vi "build_version_msg.vi"(4 "error in":errorcluster, 5 "Client version":string, 6 "Client API version":string, 7 "Response JSON":string) -> (0 "error out":errorcluster, 2 "API version":string, 3 "Message":string)   [LabVIEW 2019]
doc: "Builds a message to inform the user the compatibility between simulator and client."
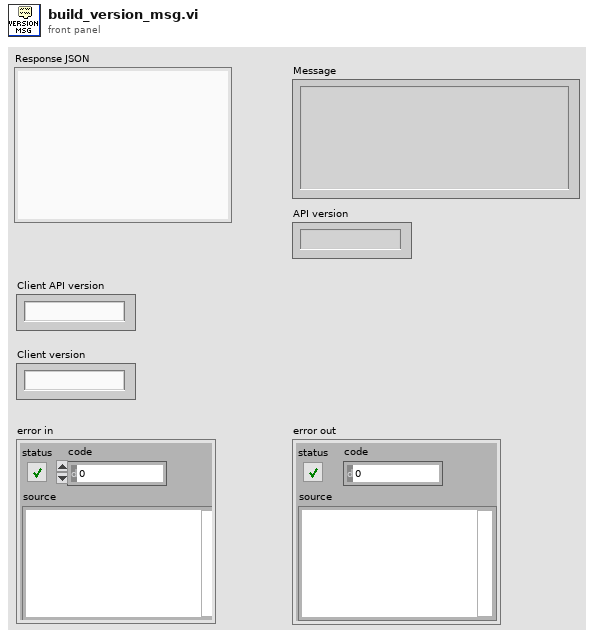
[diagram p1: front panel]
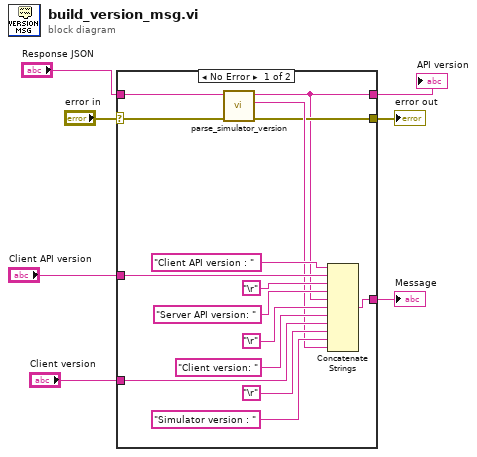
[diagram p0: block diagram]
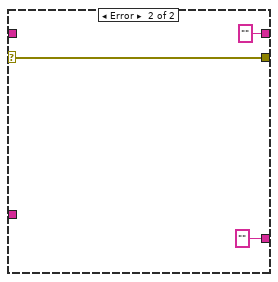
[diagram p2: hidden frame]
diagram:
  n1 = case shown="No Error" "error in" {
    selector: "error in" -> [w11 w24]
    tunnel: [w15 ""] -> w7
    tunnel: [w10 w24] -> w5
    tunnel: "Client API version" -> [w14 _]
    tunnel: "Client version" -> [w13 _]
    tunnel: "Response JSON" -> [w9 _]
    tunnel: [w8 "" ("api_version")] -> w1
    frame No Error {
      n2 = call "parse_simulator_version.vi"("error in"=w11, "Response JSON"=w9) -> ("error out"=w10:errorcluster, "Simulator version"=w12:string, "API version"=w8:string)  [unwired: 3 in]
      n3 = Concatenate Strings("Client API version : " ("string"), w14, "\r", "Server API version: " ("string"), w8, "\r", "Client version: " ("string"), w13, "\r", "Simulator version : " ("string"), w12) -> (w15:string)
    }
    frame Error {
    }
  }
  "Message" <- w7
  "error out" <- w5
  "API version" <- w1
